vi "SR830_Messgeraet.vi"(2 "refnum":refnum<file>, 3 "Numerisch":i8 min=0 max=2 step=1) -> ()   [LabVIEW 2016]
uses:
  Global/Global Variables/Data_Display_global.vi
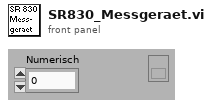
[diagram p1: front panel]
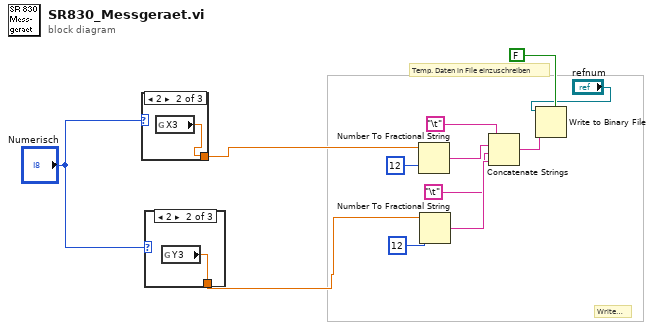
[diagram p0: block diagram]
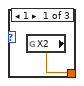
[diagram p2: hidden frame]
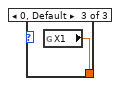
[diagram p3: hidden frame]
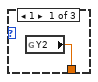
[diagram p4: hidden frame]
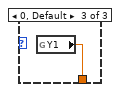
[diagram p5: hidden frame]
diagram:
  # "Temp. Daten in File einzuschreiben"
  # "Write File"
  n1 = case shown="2" "Numerisch" {
    tunnel: [w13 w14 w15] -> w3
    frame 1 {
      n2 = global read "Data_Display_global.vi" "X2"() -> (w13:dbl)
    }
    frame 2 {
      n3 = global read "Data_Display_global.vi" "X3"() -> (w14:dbl)
    }
    frame 0, Default {
      n4 = global read "Data_Display_global.vi" "X1"() -> (w15:dbl)
    }
  }
  n5 = case shown="2" "Numerisch" {
    tunnel: [w16 w17 w18] -> w4
    frame 1 {
      n6 = global read "Data_Display_global.vi" "Y2"() -> (w16:dbl)
    }
    frame 2 {
      n7 = global read "Data_Display_global.vi" "Y3"() -> (w17:dbl)
    }
    frame 0, Default {
      n8 = global read "Data_Display_global.vi" "Y1"() -> (w18:dbl)
    }
  }
  n9 = Number To Fractional String(number=w3, precision (6)=i16 12) -> (F-format string=w10:string)  [unwired: 2 in]
  n10 = Number To Fractional String(number=w4, precision (6)=i16 12) -> (F-format string=w9:string)  [unwired: 2 in]
  n11 = Concatenate Strings("\t", w10, "\t", w9) -> (w12:string)
  n12 = Write to Binary File ("Write File")(file (use dialog)="refnum", data=w12, 5:FALSE ("prepend array or string size? (T)")) -> ()  [unwired: 3 in, 3 out]
